vi "Build Config Table.vi"(8 "error in (no error)":errorcluster, 11 "Config Alert Module in":refnum<class "Config Monitor Module.lvclass">) -> (0 "error out":errorcluster, 1 "All Good":bool, 2 "Node Config Info":T1[](array[typedef]), 3 "Config Alert Module out":refnum<class "Config Monitor Module.lvclass">)   [LabVIEW 2020, in "Volatus.lvlib" / "Config Monitor Module.lvclass"]
uses:
  Config Monitor Module.lvclass
  C:/dev/lv20CE/relink/lv-volatus/Volatus/Module/Module.lvclass
  Node Config Info.ctl
  Config Monitor Module.lvclass/Config Monitor Module.ctl
  Module/Module.lvclass/Module.ctl
  VolatusAPI/Build Node URL.vi
  <vilib>/NI/Advanced HTTP Client/GET.vi
  VolatusAPI/VolatusAPI.lvclass
  ConfigInfoValue/ConfigInfoValue.lvclass
  Module/Module.lvclass
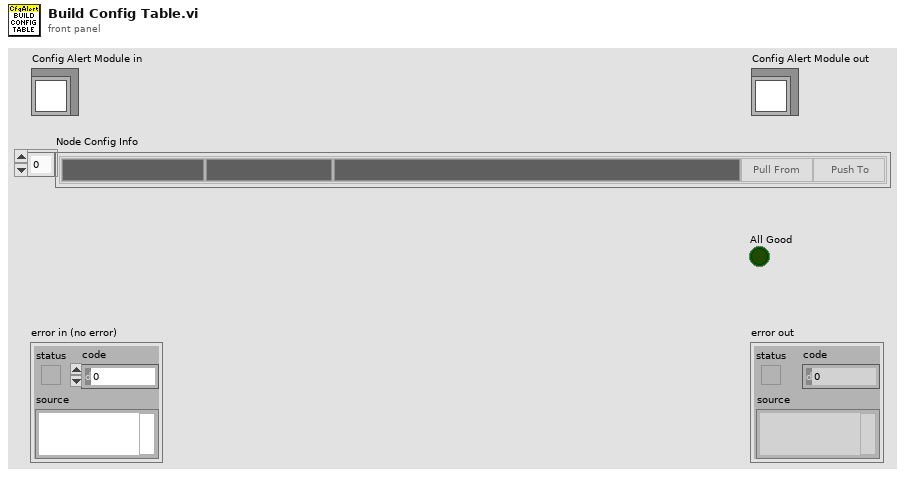
[diagram p1: front panel]
types:
  T1 = typedef "Volatus.lvlib/Config Monitor Module.lvclass/Node Config Info.ctl" = cluster{"Node":string, "Config Version":string, "Config Hash":string, "Pull":bool, "Push":bool, "Version Color":u32, "Hash Color":u32, "Node Color":u32}
  T2 = typedef "Volatus.lvlib/Config Info.ctl" = cluster{"System":string, "Cluster":string, "Node":string, "Path":path, "Version":string, "Hash":string}
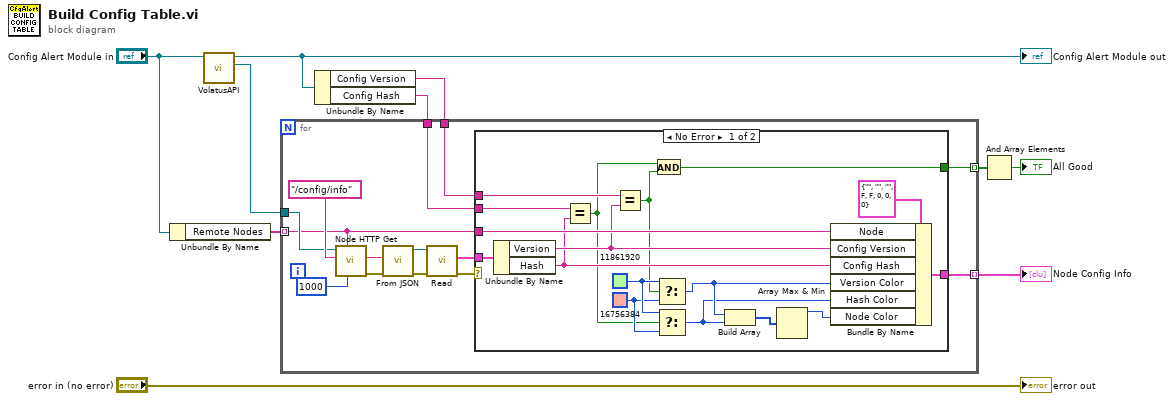
[diagram p0: block diagram]
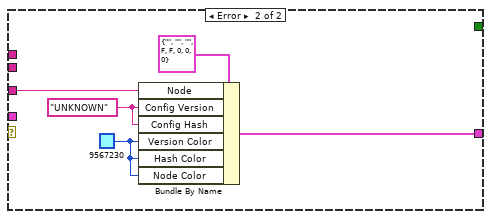
[diagram p2: hidden frame]
diagram:
  n1 = Unbundle By Name("Config Alert Module in") -> ("Remote Nodes"=w8:string[])
  n2 = call "VolatusAPI.vi"("Module in"="Config Alert Module in") -> ("VolatusAPI"=w7:refnum<class "VolatusAPI.lvclass">, "Module out"=w6:refnum<class "Config Monitor Module.lvclass">)  [unwired: 9 in]
  "Config Alert Module out" <- w6
  n3 = Unbundle By Name(w6) -> ("Config Version"=w4:string, "Config Hash"=w5:string)
  n4 = for {
    tunnel: w8 -> [w18] mode=indexing
    tunnel: w7 -> [w21]
    tunnel: w5 -> [w15]
    tunnel: w4 -> [w14]
    tunnel: [w13] -> w3 mode=indexing
    tunnel: [w12] -> w2 mode=indexing
    n5 = call "Node HTTP Get.vi"("Timeout ms (10000)"=1000, "Node Name"=w18, "Path"="/config/info", "VolatusAPI in"=w21) -> ("error out"=w20:errorcluster, "Response"=w22:string)  [unwired: 3 in, 3 out]
    n6 = call "From JSON.vi"("error in (no error)"=w20, "JSON"=w22) -> ("error out"=w17:errorcluster, "ConfigInfoValue out"=w19:refnum<class "ConfigInfoValue.lvclass">)  [unwired: 8 in]
    n7 = call "Read.vi"("ConfigInfoValue in"=w19) -> ("Config Info"=w16:T2)  [unwired: 10 in]
    n8 = case shown="No Error" w17 {
      tunnel: w18 -> [w39 w44]
      tunnel: w16 -> [w38 _]
      tunnel: [w37 w42] -> w13
      tunnel: w15 -> [w34 _]
      tunnel: w14 -> [w36 _]
      tunnel: [w28 _] -> w12
      frame No Error {
        w31 = u32 16756384 ("Version Color")
        w32 = u32 11861920 ("Version Color")
        n9 = Unbundle By Name(w38) -> ("Version"=w35:string, "Hash"=w33:string)
        n10 = Equal?(x=w34, y=w33) -> (x = y?=w29:bool)
        n11 = Equal?(x=w36, y=w35) -> (x = y?=w30:bool)
        n12 = And(x=w29, y=w30) -> (x .and. y?=w28:bool)
        n13 = Select(t=w32, s=w30, f=w31) -> (s? t:f=w27:u32)
        n14 = Select(t=w32, s=w29, f=w31) -> (s? t:f=w26:u32)
        n15 = Build Array(w27, w26) -> (w25:u32[])
        n16 = Array Max & Min(array=w25) -> (max value=w24:u32)  [unwired: 3 out]
        n17 = Bundle By Name(cluster=T1 {"Node"="", "Config Version"="", "Config Hash"="", "Pull"=FALSE, "Push"=FALSE, "Version Color"=0, "Hash Color"=0, "Node Color"=0} ("Cluster"), "Node"=w39, "Config Version"=w35, "Config Hash"=w33, "Version Color"=w27, "Hash Color"=w26, "Node Color"=w24) -> (w37:T1)
      }
      frame Error {
        w41 = u32 9567230 ("Version Color")
        w43 = "UNKNOWN" ("Config Version")
        n18 = Bundle By Name(cluster=T1 {"Node"="", "Config Version"="", "Config Hash"="", "Pull"=FALSE, "Push"=FALSE, "Version Color"=0, "Hash Color"=0, "Node Color"=0} ("Cluster"), "Node"=w44, "Config Version"=w43, "Config Hash"=w43, "Version Color"=w41, "Hash Color"=w41, "Node Color"=w41) -> (w42:T1)
      }
    }
  }
  "Node Config Info" <- w3
  n19 = And Array Elements(Boolean array=w2) -> (logical AND=→"All Good":bool)
  "error out" <- "error in (no error)"
